vi "A33ConfigureBurst_py.vi"(8 "error in (no error)":errorcluster, 10 "Instrument":string, 11 "socket in":refnum<class "zmq_socket.lvclass">) -> (0 "error out":errorcluster, 1 "Standalone":bool, 2 "resulting string":string, 3 "socket out":refnum<class "zmq_socket.lvclass">)   [LabVIEW 2022 SP3]
doc: "Selects the waveform shape, frequency, amplitude, offset, and phase for a standard waveform."
uses:
  <vilib>/addons/zeromq/zmq_socket.lvclass
panel:
  in  "Internal period":dbl=0.10000000149011612 format="%_12g"
  in  "Gate polarity (F: positive)":bool
  in  "Burst phase (-360..+360)":dbl format="%_12g"
  in  "Channel (0: Channel 1)":i32(ring) items=["Channel 1"=1, "Channel 2"=2]
  in  "Enable Burst (T: Enable)":bool=TRUE
  in  "Burst Count (1-100M)":i32=1
  in  "Burst Mode (0: Triggered)":i32(ring) items=["Triggered", "Gated"]
  # "Phase is not delay!!"
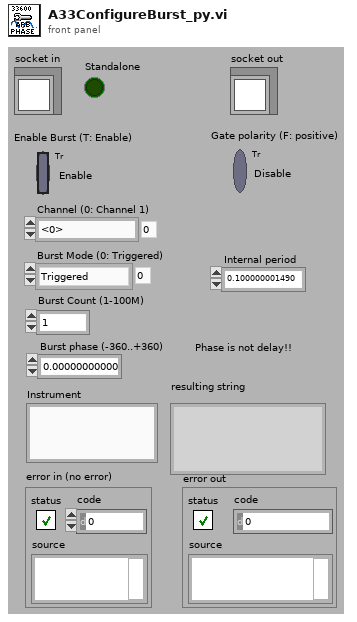
[diagram p1: front panel]
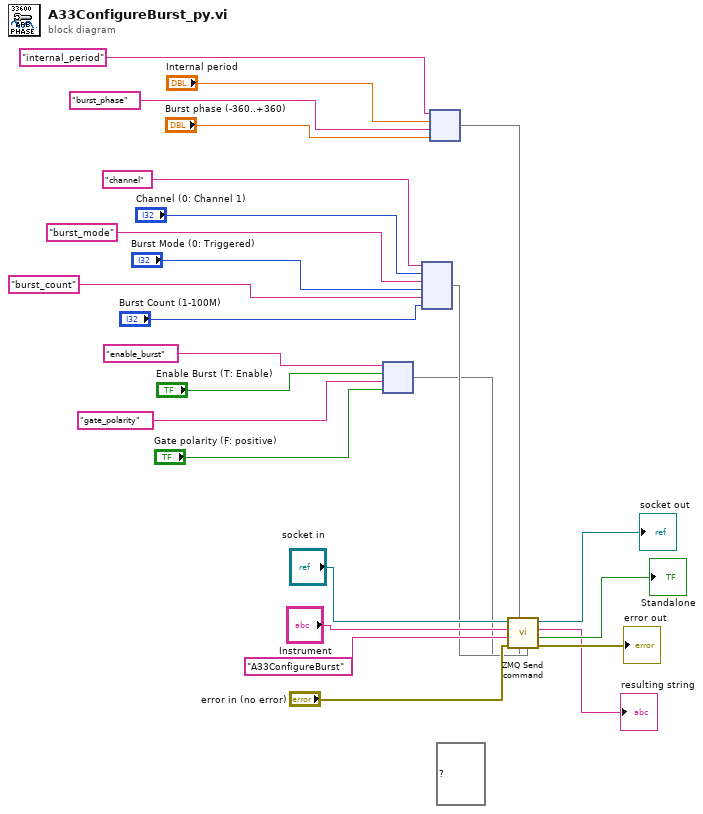
[diagram p0: block diagram]
diagram:
  (unwired) map{string, u16} {} ("map")
  n1 = node("enable_burst" ("key"), "Enable Burst (T: Enable)", "gate_polarity" ("key"), "Gate polarity (F: positive)") -> (w1:map{string, bool})
  n2 = node("channel" ("key"), "Channel (0: Channel 1)", "burst_mode" ("key"), "Burst Mode (0: Triggered)", "burst_count" ("key"), "Burst Count (1-100M)") -> (w11:map{string, i32})
  n3 = node("internal_period" ("key"), "Internal period", "burst_phase" ("key"), "Burst phase (-360..+360)") -> (w6:map{string, dbl})
  n4 = call "ZMQ Send command.vi"("Int args"=w11, "Bool args"=w1, "DBL args"=w6, "error in"="error in (no error)", "Command"="A33ConfigureBurst", "Instrument"="Instrument", "socket in"="socket in") -> ("error out"=→"error out":errorcluster, "Standalone"=→"Standalone":bool, "Recieved message"=→"resulting string":string, "socket out"=→"socket out":refnum<class "zmq_socket.lvclass">)  [unwired: 1 in]
